vi "PrePurge_Complete.vi"(0 "Data in":T1, 5 "Boiler Status Indicators":refnum<vi>, 7 "Boiler Controls":refnum<vi>, 9 "State":T2, 11 "error in (no error)":errorcluster) -> (4 "Data out":T1, 15 "error out":errorcluster)   [LabVIEW 2023]
uses:
  Controls/State.ctl
  Controls/DataCluster.ctl
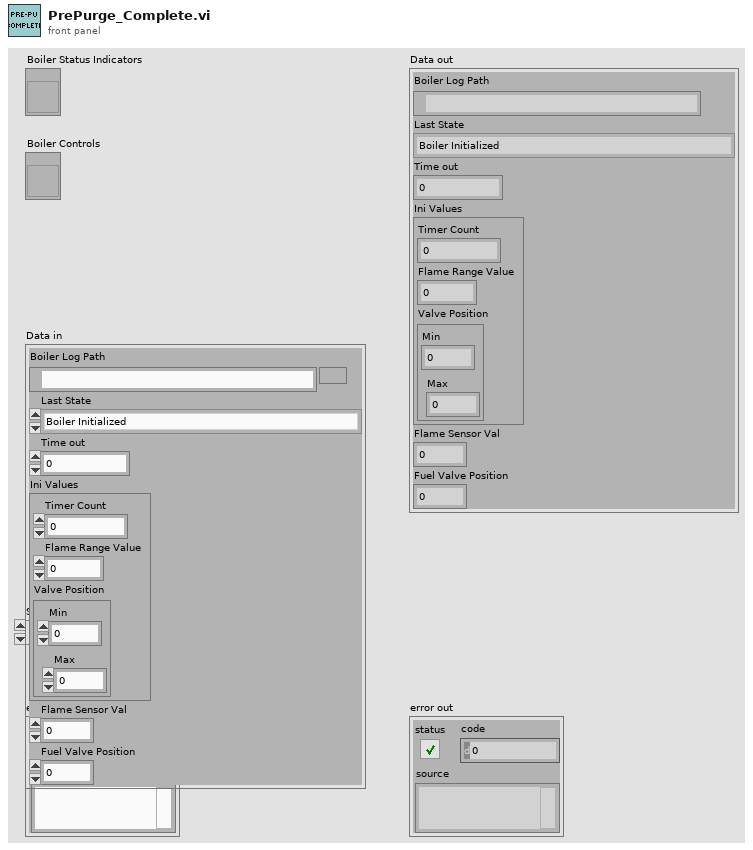
[diagram p1: front panel]
types:
  T1 = typedef "DataCluster.ctl" = cluster{"Boiler Log Path":path, "Last State":T2, "Time out":i32, "Ini Values":cluster{"Timer Count":dbl, "Flame Range Value":dbl, "Valve Position ":cluster{"Min":dbl, "Max":dbl}}, "Flame Sensor Val":dbl, "Fuel Valve Position":dbl}
  T2 = typedef "State.ctl" = enum16{"Boiler Initialized", "Boiler Ready", "Start Pre-Purge", "Pre-Purge Complete", "Pilot On", "Pilot Proved", "Force Draft Fan ON", "Boiler Running", "Start Shutdown Purge", "Shutdown Purge Complete", "Wait for Something"}
  T3 = typedef "Boiler Status Indicators.ctl" = cluster{"Status":string, "Primary Fan":bool, "Natural Gas Valve":bool, "Pilot":bool, "Fuel Valve":bool, "Forced Draft Fan":bool, "Time Count":dbl}
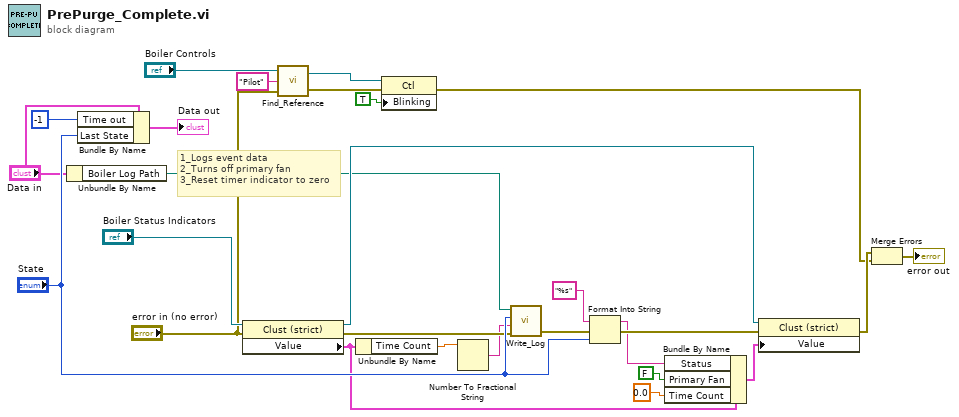
[diagram p0: block diagram]
diagram:
  # "1_Logs event data\n2_Turns off primary fan\n3_Reset timer indicator to zero"
  n1 = Unbundle By Name("Data in") -> ("Boiler Log Path"=w12:path)
  n2 = Bundle By Name(cluster="Data in", "Time out"=-1, "Last State"="State") -> (→"Data out":T1)
  n3 = property class="Clust (strict)"(reference="Boiler Status Indicators", error in="error in (no error)") -> (reference out=w17:refnum<vi>, error out=w15:errorcluster, "Value"=w19:T3)
  n4 = call "Find_Reference.vi"("error in (no error)"="error in (no error)", "Label"="Pilot", "Cluster in"="Boiler Controls") -> ("error out"=w7:errorcluster, "Ctl Refnum"=w6:refnum<vi>)  [unwired: 1 in]
  n5 = Unbundle By Name(w19) -> ("Time Count"=w13:dbl)
  n6 = property class="Ctl"(reference=w6, error in=w7, "Blinking"=TRUE) -> (error out=w3:errorcluster)  [unwired: 1 out]
  n7 = Number To Fractional String(number=w13) -> (F-format string=w14:string)  [unwired: 3 in]
  n8 = call "Write_Log.vi"("error in (no error)"=w15, "Event data string"=w14, "State"="State", "dup path"=w12) -> ("error out"=w23:errorcluster)  [unwired: 2 in]
  n9 = Format Into String(format string="%s", error in=w23, "State") -> (resulting string=w21:string, error out=w22:errorcluster)  [unwired: 1 in]
  n10 = Bundle By Name(cluster=w19, "Status"=w21, "Primary Fan"=FALSE, "Time Count"=0.0) -> (w20:T3)
  n11 = property class="Clust (strict)"(reference=w17, error in=w22, "Value"=w20) -> (error out=w16:errorcluster)  [unwired: 1 out]
  n12 = Merge Errors(w16, w3) -> (→"error out":errorcluster)
